vi "obliczOdleglosciZListyPunktow.vi"() -> ()   [LabVIEW 2014]
uses:
  test/testujPunktyVIs/Odleglosc.ctl
  glownaMaszynaStanowVIs/wczytajListePunktowVIs/RodzajPomiarow.ctl
panel:
  out "Odleglosci":T1[][](array[typedef]) {"Odległość [m]" format="%#.2g"}
  in  "Promień [m]":dbl=1.0 format="%#_13g"
  in  "Minimalna odległość":dbl=0.7 format="%#_13g"
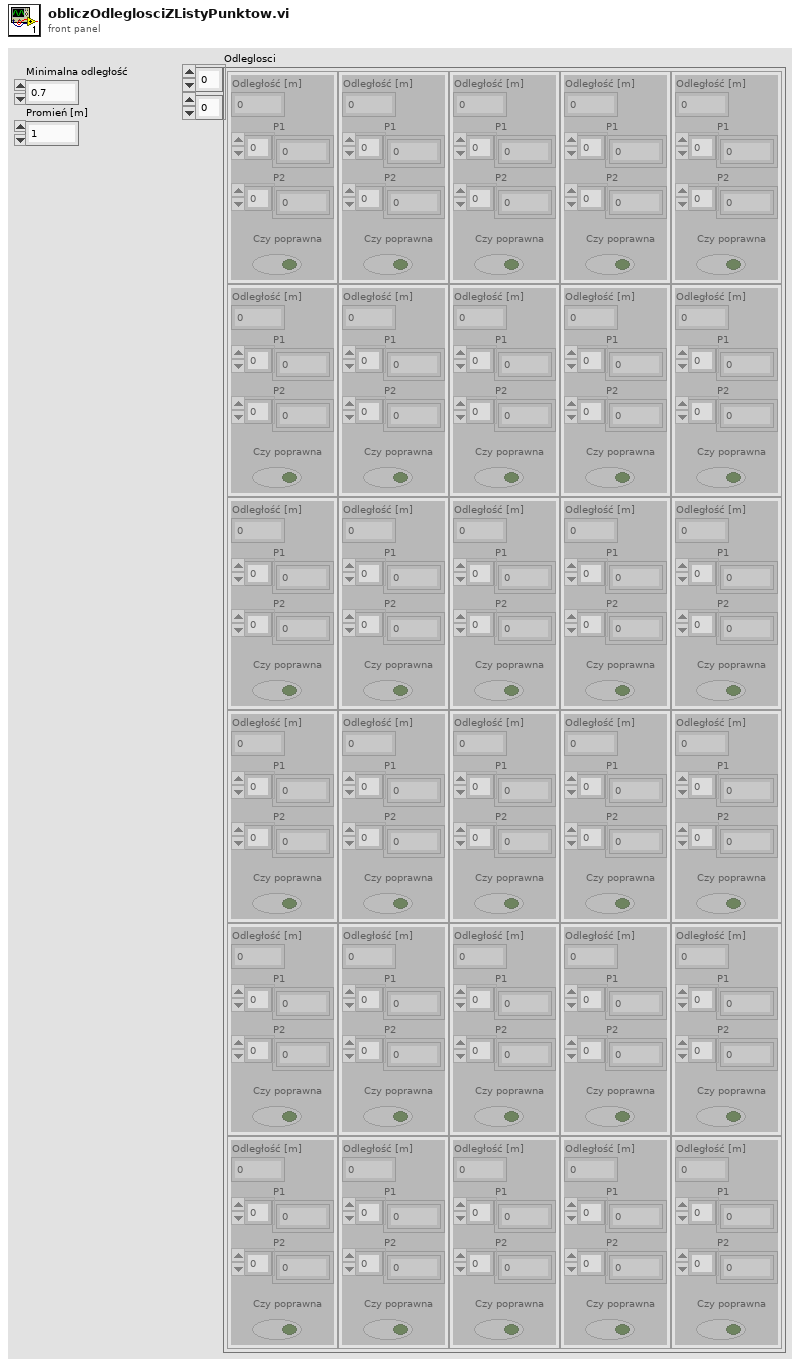
[diagram p1: front panel]
types:
  T1 = typedef "Odleglosc.ctl" = cluster{"Odległość [m]":dbl, "P1":i32[], "P2":i32[], "Czy poprawna":bool}
  T2 = typedef "RodzajPomiarow.ctl" = enum16{"Izolacyjność Akustyczna ISO 10140", "Sekwencja testowa", "Definicja użytkownika"}
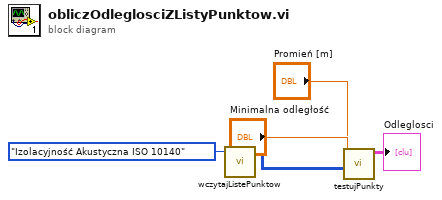
[diagram p0: block diagram]
diagram:
  n1 = call "wczytajListePunktow.vi"("Rodzaj pomiarow"=RodzajPomiarow."Izolacyjność Akustyczna ISO 10140") -> ("Wspolrzedne katowe"=w4:i32[][])  [unwired: 4 in]
  n2 = call "testujPunkty.vi"("Punkty"=w4, "Minimalna odległość"="Minimalna odległość", "Promień [m]"="Promień [m]") -> ("Odleglosci"=→"Odleglosci":T1[][])  [unwired: 8 in]
